vi "Datalog Parsing Program - For Non-Labview Users to get .bin data packing.vi"() -> ()   [LabVIEW 2014]
uses:
  ATS-VI/ATS_ctl/ExtTrigRange.ctl
  ATS-VI/ATS_ctl/Coupling.ctl
  ATS-VI/ATS_ctl/ExtTrigger.ctl
  ATS-VI/ATS_ctl/TriggerEngine.ctl
  ATS-VI/ATS_ctl/TriggerOperation.ctl
  ATS-VI/ATS_ctl/Trigger.ctl
  ATS-VI/ATS_ctl/Bandwidth.ctl
  ATS-VI/ATS_ctl/Impedance.ctl
  ATS-VI/ATS_ctl/Range.ctl
  ATS-VI/ATS_ctl/InputCtrl.ctl
  ATS-VI/ATS_ctl/ClockEdge.ctl
  ATS-VI/ATS_ctl/ClockRate.ctl
  ATS-VI/ATS_ctl/ClockSource.ctl
  ATS-VI/ATS_ctl/Clock.ctl
  ATS-VI/ATS_ctl/Record.ctl
  ATS-VI/ATS_ctl/ATS_Global.ctl
  Classes/Galvo/Scanning Cluster.ctl
  Classes/Galvo/Galvo.lvclass
panel:
  out "output cluster":cluster{"Length":u32, "A/B":u32, "B-Scan":u32}
  out "record(s)":cluster{"Scanning":T1, "Setup_In":T2}[](array[cluster]) {"Scanning"."Fast Axis Amp" max=20 format="%#.2f"; "Scanning"."Slow Axis Amp" max=20 format="%#.2f"; "Scanning"."Slow Axis Offset" max=10 format="%#.2f"; "Scanning"."Fast Axis Offset" max=10 format="%#.2f"; "Setup_In"."Clock"."ClckEdge" items=["Rising", "Falling"]; "Setup_In"."Clock"."ClckRate" items=["1 kS/s", "2 kS/s", "5 kS/s", "10 kS/s", "20 kS/s", "50 kS/s", "100 kS/s", "200 kS/s", "500 kS/s", "1 MS/s", "2 MS/s", "5 MS/s", "10 MS/s", "20 MS/s", "25 MS/s", "50 MS/s", "100 MS/s", "125 MS/s", "200 MS/s", "250 MS/s", "500 MS/s", "1 GS/s"]; "Setup_In"."Input B"."Range" items=["20mv", "40mV", "50mV", "80mV", "100mV", "200mV", "400mV", "500mV", "800mV", "1 V", "2 V", "4 V", "5 V", "8 V", "10 V", "20 V"]; "Setup_In"."Trigger"."Timeout (s)" format="%.2f"; "Setup_In"."Input A"."Range" items=["20mv", "40mV", "50mV", "80mV", "100mV", "200mV", "400mV", "500mV", "800mV", "1 V", "2 V", "4 V", "5 V", "8 V", "10 V", "20 V"]}
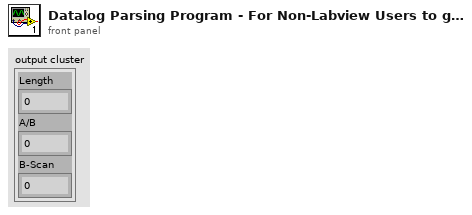
[diagram p1: front panel]
types:
  T1 = typedef "Galvo.lvclass/Scanning Cluster.ctl" = cluster{"Fast Axis Offset":sgl, "Slow Axis Offset":sgl, "Slow Axis Amp":sgl, "Fast Axis Amp":sgl, "Scan Pattern":enum16{"Raster"}}
  T2 = typedef "ATS_Global.ctl" = cluster{"Record":T3, "Clock":T4, "Input A":T8, "Input B":T8, "Trigger":T13}
  T3 = typedef "Record.ctl" = cluster{"Count":u32, "Presize":u32, "Length":u32}
  T4 = typedef "Clock.ctl" = cluster{"ClckSource":T5, "ClckRate":T6, "ClckEdge":T7, "Decimation":u32}
  T5 = typedef "ClockSource.ctl" = enum16{"Internal", "External", "Medium Ext.", "Slow Ext.", "Ext. AC", "Ext. DC", "Ext. (PLL)"}
  T6 = typedef "ClockRate.ctl" = u32
  T7 = typedef "ClockEdge.ctl" = u16
  T8 = typedef "InputCtrl.ctl" = cluster{"Coupling":T9, "Range":T10, "Impedance":T11, "Bandwidth":T12}
  T9 = typedef "Coupling.ctl" = enum16{"AC", "DC"}
  T10 = typedef "Range.ctl" = u32
  T11 = typedef "Impedance.ctl" = enum16{"1M ohms", "50 ohms"}
  T12 = typedef "Bandwidth.ctl" = enum16{"Full Bandwidth", "Reduce Bandwidth"}
  T13 = typedef "Trigger.ctl" = cluster{"TrigOperation":T14, "Timeout (s)":dbl, "Trig. Delay":u32, "Engine X":T15, "Engine Y":T15, "ExtTrigControl":T16}
  T14 = typedef "TriggerOperation.ctl" = enum16{"Only X", "Only Y", "X or Y", "X and Y", "X xor Y", "X and not Y", "not X and Y"}
  T15 = typedef "TriggerEngine.ctl" = cluster{"Source":enum32{"Chan_A", "Chan_B", "External", "Disable"}, "Slope":enum32{"Positive", "Negative"}, "Level":u32}
  T16 = typedef "ExtTrigger.ctl" = cluster{"Coupling":T9, "Range":T17}
  T17 = typedef "ExtTrigRange.ctl" = enum16{"1 V", "5 V", "TTL"}
  T18 = typedef "Galvo.lvclass/Scanning Cluster.ctl" = cluster{"Fast Axis Offset":sgl, "Slow Axis Offset":sgl, "Slow Axis Amp":sgl, "Fast Axis Amp":sgl, "B-scans (rings)":u32, "A(cluster)/B":u32, "Scan Pattern":enum16{"Raster"}}
  T19 = cluster{"Length":u32, "A(cluster)/B":u32, "B-scans (rings)":u32}
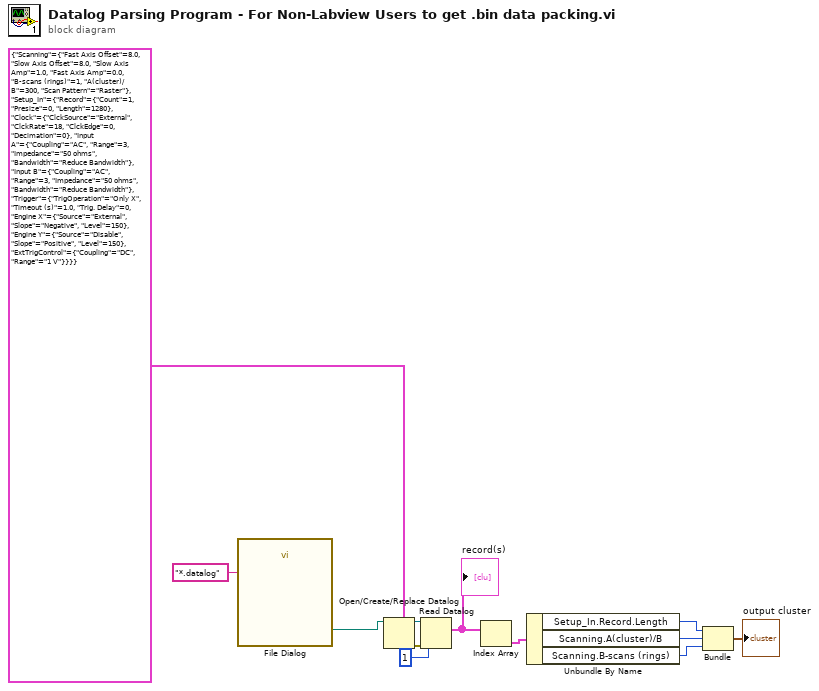
[diagram p0: block diagram]
diagram:
  n1 = call "File Dialog"("pattern (all files)"="*.datalog") -> ("selected path"=w11:path)  [unwired: 11 in, 3 out]
  n2 = Open/Create/Replace Datalog(5:cluster{"Scanning":T18, "Setup_In":T2} {"Scanning"={"Fast Axis Offset"=8.0, "Slow Axis Offset"=8.0, "Slow Axis Amp"=1.0, "Fast Axis Amp"=0.0, "B-scans (rings)"=1, "A(cluster)/B"=300, "Scan Pattern"=enum."Raster"}, "Setup_In"={"Record"={"Count"=1, "Presize"=0, "Length"=1280}, "Clock"={"ClckSource"=enum."External", "ClckRate"=18, "ClckEdge"=0, "Decimation"=0}, "Input A"={"Coupling"=enum."AC", "Range"=3, "Impedance"=enum."50 ohms", "Bandwidth"=enum."Reduce Bandwidth"}, "Input B"={"Coupling"=enum."AC", "Range"=3, "Impedance"=enum."50 ohms", "Bandwidth"=enum."Reduce Bandwidth"}, "Trigger"={"TrigOperation"=enum."Only X", "Timeout (s)"=1.0, "Trig. Delay"=0, "Engine X"={"Source"=enum."External", "Slope"=enum."Negative", "Level"=150}, "Engine Y"={"Source"=enum."Disable", "Slope"=enum."Positive", "Level"=150}, "ExtTrigControl"={"Coupling"=enum."DC", "Range"=enum."1 V"}}}} ("Sampling Info"), 11:w11) -> (0:w10:errorcluster, 3:w9:refnum<k1>)  [unwired: 4 in, 1 out]
  n3 = Read Datalog(4:w10, 6:1 ("count (1)"), 7:w9) -> (2:w6:cluster{"Scanning":T18, "Setup_In":T2}[])  [unwired: 2 out]
  "record(s)" <- w6
  n4 = Index Array(array=w6) -> (element=w5:cluster{"Scanning":T18, "Setup_In":T2})  [unwired: 1 in]
  n5 = Unbundle By Name(w5) -> ("Setup_In.Record.Length"=w4:u32, "Scanning.A(cluster)/B"=w3:u32, "Scanning.B-scans (rings)"=w2:u32)
  n6 = Bundle("Length"=w4, "A(cluster)/B"=w3, "B-scans (rings)"=w2) -> (→"output cluster":T19)  [unwired: 1 in]
